vi "isDelayLabel.vi"(8 "error in (no error)":errorcluster, 11 "ScriptEvent in":refnum<class "ScriptEvent.lvclass">) -> (0 "error out":errorcluster, 2 "delay":bool, 3 "ScriptEvent out":refnum<class "ScriptEvent.lvclass">)   [LabVIEW 2011, in "Tools.lvlib" / "Scripting.lvlib" / "ScriptEvent.lvclass"]
uses:
  ScriptEvent.lvclass
  Delay/Delay.lvclass
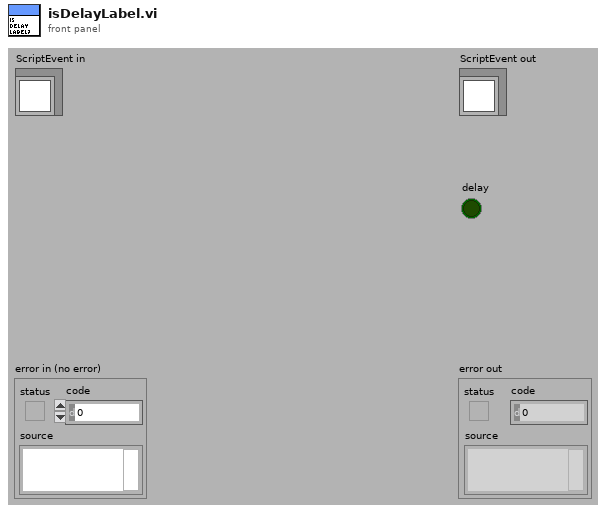
[diagram p1: front panel]
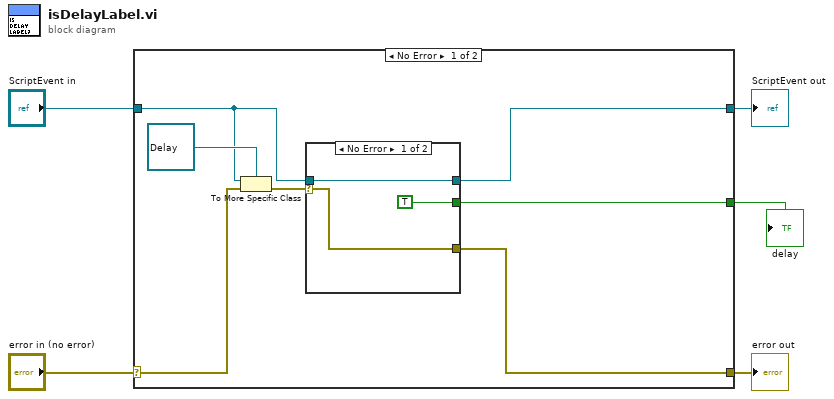
[diagram p0: block diagram]
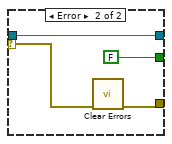
[diagram p2: hidden frame]
diagram:
  n1 = case shown="No Error" "error in (no error)" {
    selector: "error in (no error)" -> [w11 w21]
    tunnel: [w7 w21] -> w4
    tunnel: [w8 w20] -> w2
    tunnel: "ScriptEvent in" -> [w6 w20]
    tunnel: [w9 _] -> w1
    frame No Error {
      n2 = To More Specific Class(target class=refnum<class "Delay.lvclass"> refnum ("Tools.lvlib:Scripting.lvlib:Delay.lvclass"), reference=w6, error in=w11) -> (error out=w10:errorcluster)  [unwired: 1 out]
      n3 = case shown="No Error" w10 {
        selector: w10 -> [w13 w16]
        tunnel: w6 -> [w14 w18]
        tunnel: [TRUE FALSE] -> w9
        tunnel: [w14 w18] -> w8
        tunnel: [w13 w17] -> w7
        frame No Error {
        }
        frame Error {
          n4 = call <vilib>:"Clear Errors.vi"("error in (no error)"=w16) -> ("error out"=w17:errorcluster)  [unwired: 6 in]
        }
      }
    }
    frame Error {
    }
  }
  "error out" <- w4
  "ScriptEvent out" <- w2
  "delay" <- w1
